vi "Get Ultimus V Total Status.vi"(0 "VISA resource name":refnum<visa-resource-name>, 11 "error in (no error)":errorcluster) -> (2 "AI Mode Status":string, 3 "AI Mode Function":string, 4 "VISA resource name out":refnum<visa-resource-name>, 6 "Trigger Value":dbl, 8 "Current Timer/Counter Value":dbl, 10 "Dispense Mode":string, 13 "AI End Address":i32, 14 "AI Start Address":i32, 15 "error out":errorcluster)   [LabVIEW 2018, in "EFD Ultimus V.lvlib"]
doc: "Returns the status and values of the Auto Increment mode as well as the dispense mode. 'D0' is the number zero (0).\n\nHost Format: AU---\n\nReturn Format: D0AIiMmSssssDdddddddVIqVvvvvIttttTMxSAaaaEeee\n i: Auto Increment mode status. 0 = Off, 1 = Enabled\n m: Auto Increment mode function. 1 = Timer, 2 = Count\nssss: Trigger Value. \nddddddd: Current Timer/Counter value\nq: Defaulted to 0\nvvvv: Defaulted to 0001\ntttt: Defaulted to 0001\n x: Dispense mode. 0 = Timed, 1 = Steady, 2 = Teach\naaa: Auto Increment Start Address. 000 - 399\neee: Auto Increment End Address. 000 - 399"
uses:
  EFD Ultimus V.lvlib
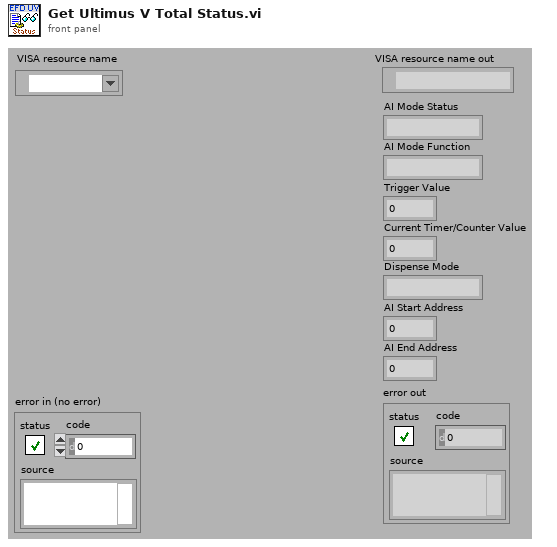
[diagram p1: front panel]
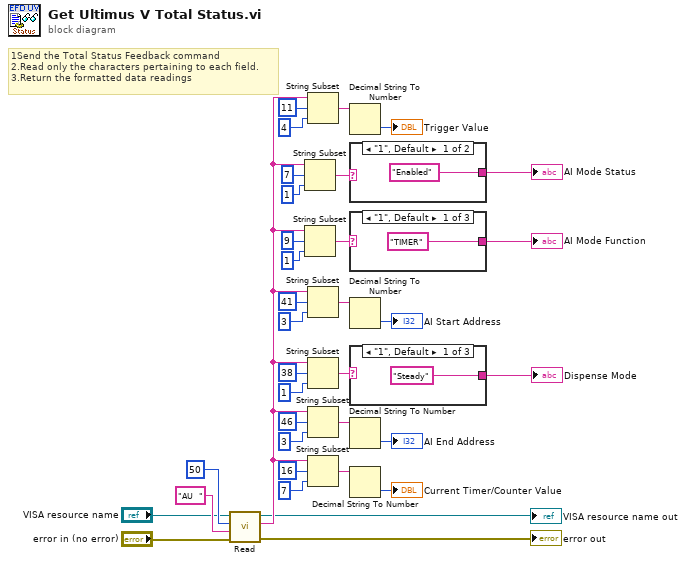
[diagram p0: block diagram]
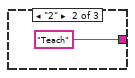
[diagram p2: hidden frame]
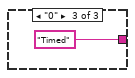
[diagram p3: hidden frame]
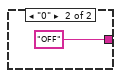
[diagram p4: hidden frame]
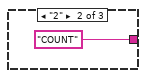
[diagram p5: hidden frame]
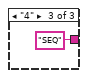
[diagram p6: hidden frame]
diagram:
  # "1Send the Total Status Feedback command\n2.Read only the characters pertaining to each field.\n3.Return the formatted data readings"
  n1 = call "Read.vi"("error in (no error)"="error in (no error)", "Command To Write"="AU  ", "Bytes to Read (11)"=u32 50 ("Bytes to Read from Buffer"), "VISA resource name"="VISA resource name") -> ("error out"=→"error out":errorcluster, "Ultimus V Feedback Data"=w15:string, "VISA resource name out"=→"VISA resource name out":refnum<visa-resource-name>)  [unwired: 5 out]
  n2 = String Subset(string=w15, offset (0)=7, length (rest)=1 ("length (rest)")) -> (substring=w32:string)
  n3 = String Subset(string=w15, offset (0)=9, length (rest)=1 ("length (rest)")) -> (substring=w30:string)
  n4 = String Subset(string=w15, offset (0)=11, length (rest)=4 ("length (rest)")) -> (substring=w8:string)
  n5 = String Subset(string=w15, offset (0)=41, length (rest)=3 ("length (rest)")) -> (substring=w10:string)
  n6 = String Subset(string=w15, offset (0)=38, length (rest)=1 ("length (rest)")) -> (substring=w34:string)
  n7 = String Subset(string=w15, offset (0)=46, length (rest)=3 ("length (rest)")) -> (substring=w6:string)
  n8 = String Subset(string=w15, offset (0)=16, length (rest)=7 ("length (rest)")) -> (substring=w4:string)
  n9 = Decimal String To Number(string=w8) -> (number=→"Trigger Value":i32)  [unwired: 3 out]
  n10 = case shown="\"1\", Default" w32 {
    tunnel: ["Enabled" ("Trigger Value") "OFF" ("Trigger Value")] -> w33
    frame "1", Default {
    }
    frame "0" {
    }
  }
  "AI Mode Status" <- w33
  n11 = case shown="\"1\", Default" w30 {
    tunnel: ["TIMER" ("Trigger Value") "COUNT" ("Trigger Value") "SEQ" ("Trigger Value")] -> w31
    frame "1", Default {
    }
    frame "2" {
    }
    frame "4" {
    }
  }
  "AI Mode Function" <- w31
  n12 = Decimal String To Number(string=w10) -> (number=→"AI Start Address":i32)  [unwired: 3 out]
  n13 = case shown="\"1\", Default" w34 {
    tunnel: ["Steady" ("Trigger Value") "Teach" ("Trigger Value") "Timed" ("Trigger Value")] -> w35
    frame "1", Default {
    }
    frame "2" {
    }
    frame "0" {
    }
  }
  "Dispense Mode" <- w35
  n14 = Decimal String To Number(string=w6) -> (number=→"AI End Address":i32)  [unwired: 3 out]
  n15 = Decimal String To Number(string=w4) -> (number=→"Current Timer/Counter Value":i32)  [unwired: 3 out]
